vi "NavX Background Loop.vi"() -> ()   [LabVIEW 2014]
uses:
  Global Objects.vi
  navX Library v2/navX Library v2.lvlib
panel:
  out "Yaw":dbl
  out "heading":dbl
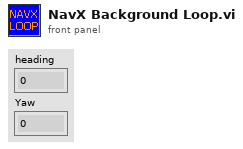
[diagram p1: front panel]
types:
  T1 = typedef "NaxX Info.ctl" = cluster{"navX Device":T2, "Current Yaw":dbl, "Active":bool}
  T2 = typedef "navX Library v2.lvlib/Z900_navX_DeviceTypeDef.ctl" = cluster{"Interface":cluster{"Protocol":T3, "Update Rate (4Hz-60Hz)":u8, "navX Open TypeDef":variant}, "Notify Packet":refnum<notifier>, "Loop VI Refnum":refnum<vi>, "Ready to Close Occurrence Refnum":refnum<k4>}
  T3 = typedef "navX Library v2.lvlib/Z900_navX_ProtocolTypeDef.ctl" = enum16{"SERIAL", "I2C", "SPI"}
  T4 = cluster{"Yaw":dbl, "Roll":dbl, "Pitch":dbl, "Heading":dbl, "Fused Heading":dbl}
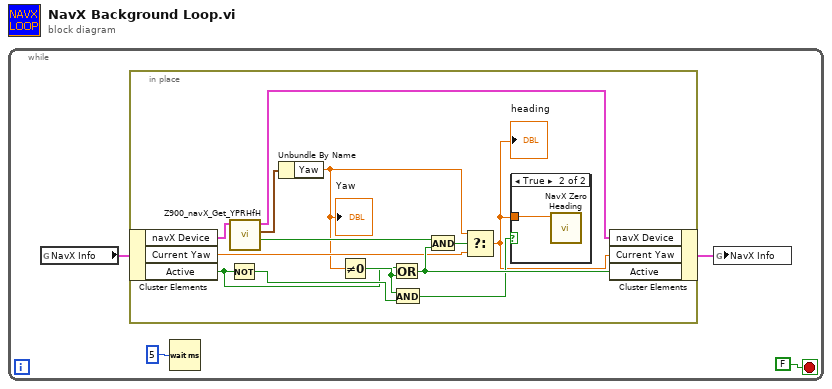
[diagram p0: block diagram]
diagram:
  n1 = while {
    stop <- FALSE stop-if-true
    n2 = global read "Global Objects.vi" "NavX Info"() -> (w4:T1)
    n3 = in-place {
      n4 = in-place-cluster #1(w4) -> ("navX Device"=w17:T2, "Current Yaw"=w12:dbl, "Active"=w8:bool)
      n5 = Not(x=w8) -> (.not. x?=w9:bool)
      n6 = call "Z900_navX_Get_YPRHfH.vi"("navX Device"=w17) -> ("Connected"=w13:bool, "YRPHfH"=w15:T4, "navX Device"=w16:T2)  [unwired: 7 in, 1 out]
      n7 = Unbundle By Name(w15) -> ("Yaw"=w5:dbl)
      "Yaw" <- w5
      n8 = Not Equal To 0?(x=w5) -> (x != 0?=w10:bool)
      n9 = Or(x=w8, y=w10) -> (x .or. y?=w14:bool)
      n10 = And(x=w10, y=w9) -> (x .and. y?=w7:bool)
      n11 = And(x=w13, y=w14) -> (x .and. y?=w11:bool)
      n12 = Select(t=w5, s=w11, f=w12) -> (s? t:f=w6:dbl)
      "heading" <- w6
      n13 = case shown="True" w7 {
        tunnel: w6 -> [_ w18]
        frame False {
        }
        frame True {
          n14 = call "NavX Zero Heading.vi"("Default Heading"=w18) -> ()  [unwired: 10 in, 1 out]
        }
      }
      n15 = in-place-cluster #1("navX Device"=w16, "Current Yaw"=w6, "Active"=w14) -> (w1:T1)
    }
    n16 = Wait (ms)(milliseconds to wait=u32 5) -> ()  [unwired: 1 out]
    n17 = global write "Global Objects.vi" "NavX Info"(w1) -> ()
  }
